vi "DataStream_RT_Send Reset.vi"(8 "Error":errorcluster, 9 "Timeout":i32=1000, 11 "Stream Writer Ref":T1) -> (0 "Error Out":errorcluster, 2 "Timed Out? Out":bool, 3 "Stream Writer Ref Out":T1)   [LabVIEW 2020]
uses:
  TypeDefs/Cluster_DataStream_RT Writer Refs.ctl
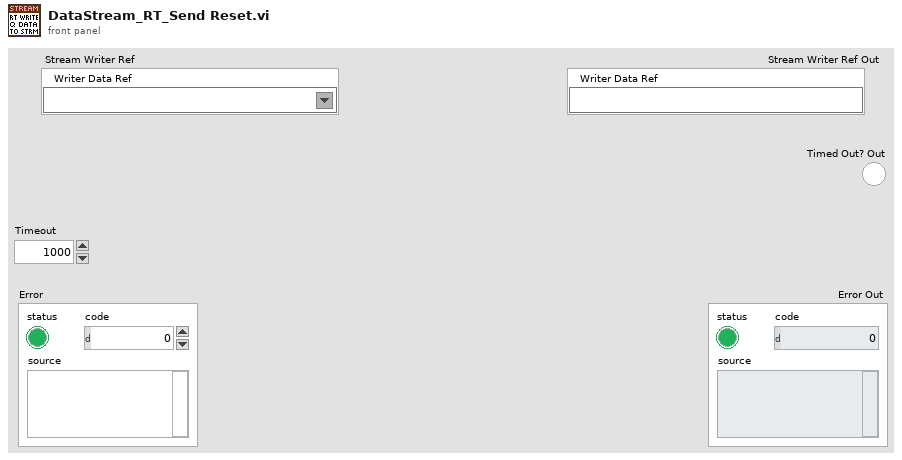
[diagram p1: front panel]
types:
  T1 = typedef "Cluster_DataStream_RT Writer Refs.ctl" = cluster{"Writer Data Ref":refnum<k21>}
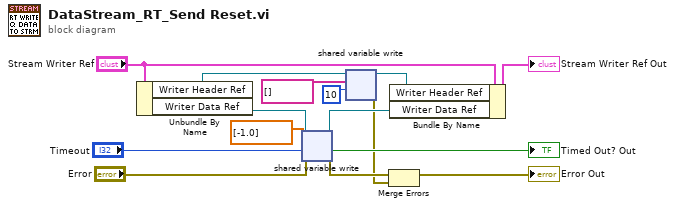
[diagram p0: block diagram]
diagram:
  n1 = Unbundle By Name("Stream Writer Ref") -> ("Writer Header Ref"=w10:refnum<k21>, "Writer Data Ref"=w9:refnum<k21>)
  n2 = shared-variable-write(w9, "Error", dbl[] [-1.0] ("data in"), "Timeout") -> (w14:refnum<k21>, w6:errorcluster, →"Timed Out? Out":bool)
  n3 = shared-variable-write(w10, string[] [] ("data in"), 10 ("timeout ms (-1)")) -> (w13:refnum<k21>, w5:errorcluster)  [unwired: 1 in, 1 out]
  n4 = Merge Errors(w6, w5) -> (→"Error Out":errorcluster)
  n5 = Bundle By Name(cluster="Stream Writer Ref", "Writer Header Ref"=w13, "Writer Data Ref"=w14) -> (→"Stream Writer Ref Out":T1)
